vi "Preview from Control.vi"(8 "error in (no error)":errorcluster, 10 "Ctl Refnum":refnum<vi>, 11 "Editor in":refnum<class "Editor.lvclass">) -> (0 "error out":errorcluster, 3 "Editor out":refnum<class "Editor.lvclass">)   [LabVIEW 2020, in "VolatusGUIEditor.lvlib" / "Editor.lvclass"]
uses:
  Editor.lvclass
  Editor.lvclass/Editor.ctl
  VolatusGUIEditor.lvlib
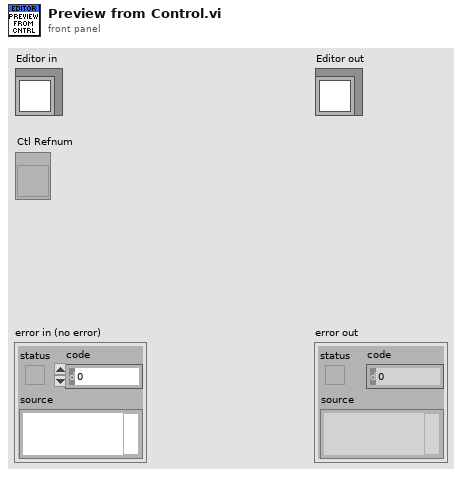
[diagram p1: front panel]
types:
  T1 = typedef "imagedata.ctl" = cluster{"image type":i32, "image depth":i32, "image":u8[], "mask":u8[], "colors":u32[], "Rectangle":cluster{"left":i16, "top":i16, "right":i16, "bottom":i16}}
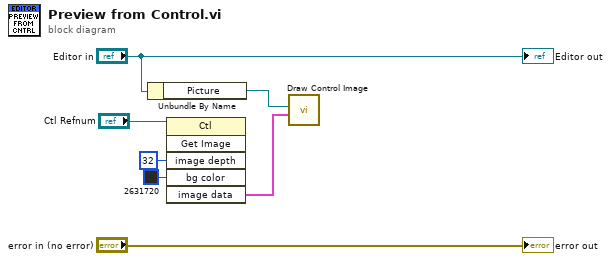
[diagram p0: block diagram]
diagram:
  n1 = Unbundle By Name("Editor in") -> ("Picture"=w2:refnum<vi>)
  n2 = invoke class="Ctl" method="Get Image"(reference="Ctl Refnum", "image depth"=32 ("Image Depth"), "bg color"=u32 2631720 ("Background Color")) -> ("image data"=w1:T1)  [unwired: 3 in, 5 out]
  n3 = call "Draw Control Image.vi"("Image"=w1, "Picture Ref"=w2) -> ()  [unwired: 10 in]
  "error out" <- "error in (no error)"
  "Editor out" <- "Editor in"
